vi "Create Header Content Class.vi"(8 "error in (no error)":errorcluster, 11 "Save Image in":refnum<class "Save Image.lvclass">) -> (0 "error out":errorcluster, 3 "Save Image out":refnum<class "Save Image.lvclass">)   [LabVIEW 2018, in "Save Image.lvclass"]
uses:
  Save Image.lvclass
  Save Image.lvclass/Save Image.ctl
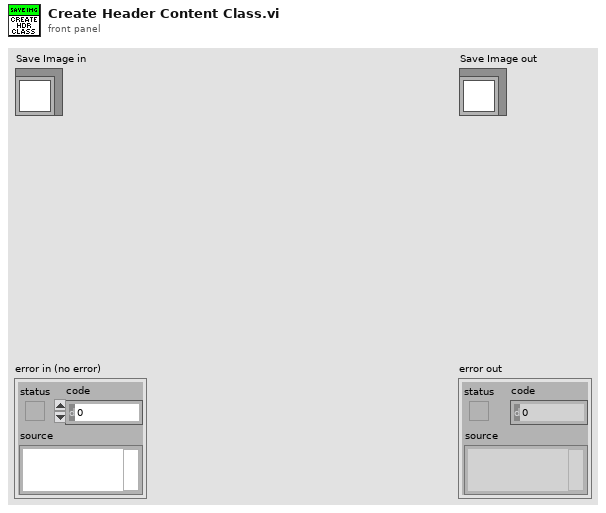
[diagram p1: front panel]
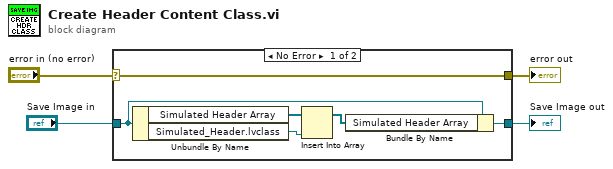
[diagram p0: block diagram]
diagram:
  n1 = case shown="No Error" "error in (no error)" {
    selector: "error in (no error)" -> [w7 w12]
    tunnel: [w7 w12] -> w3
    tunnel: [w9 w11] -> w1
    tunnel: "Save Image in" -> [w10 w11]
    frame No Error {
      n2 = Unbundle By Name(w10) -> ("Simulated Header Array"=w6:refnum<class "Simulated_Header.lvclass">[], "Simulated_Header.lvclass"=w5:refnum<class "Simulated_Header.lvclass">)
      n3 = Insert Into Array(array=w6, new element=w5) -> (w8:refnum<class "Simulated_Header.lvclass">[])  [unwired: 1 in]
      n4 = Bundle By Name(cluster=w10, "Simulated Header Array"=w8) -> (w9:refnum<class "Save Image.lvclass">)
    }
    frame Error {
    }
  }
  "error out" <- w3
  "Save Image out" <- w1
